vi "FFT-AxisVectorsFor2D.vi"(9 "Ny in":i32, 10 "Nx in":i32) -> (0 "Fy-Vector":dbl[](array[numeric]), 1 "Ny fft":i32, 2 "Fx Vector":dbl[](array[numeric]), 3 "Nx fft":i32)   [LabVIEW 2015]
uses:
  <vilib>/Analysis/1siggen.llb/Ramp Pattern by Delta.vi
  <vilib>/Analysis/NI_AALBase.lvlib
panel:
  in  "FFT shift?":bool=TRUE
  # "This creates so far only fake vector, but they have the same range and their length is correct"
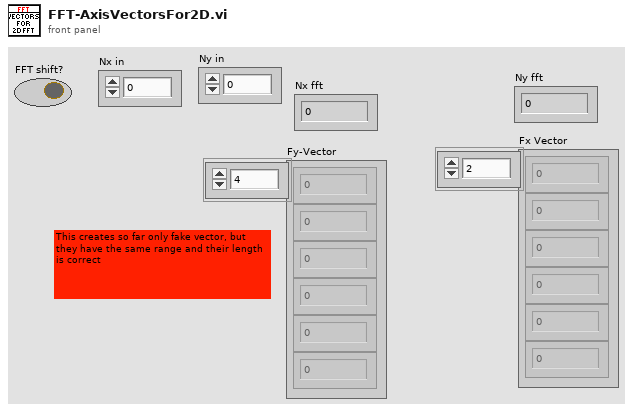
[diagram p1: front panel]
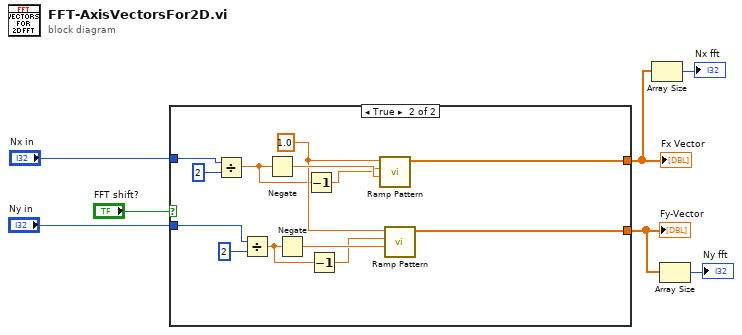
[diagram p0: block diagram]
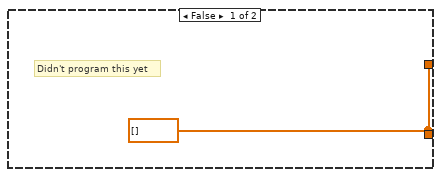
[diagram p2: hidden frame]
diagram:
  n1 = case shown="True" "FFT shift?" {
    tunnel: [w8 w21] -> w4
    tunnel: [w8 w20] -> w1
    tunnel: "Nx in" -> [_ w17]
    tunnel: "Ny in" -> [_ w19]
    frame False {
      w8 = dbl[] [] ("Ramp Pattern")
      # "Didn't program this yet"
    }
    frame True {
      w14 = 1.0 ("delta")
      n2 = Divide(x=w17, y=2) -> (x/y=w10:dbl)
      n3 = Divide(x=w19, y=2) -> (x/y=w12:dbl)
      n4 = Negate(x=w10) -> (-x=w15:dbl)
      n5 = Negate(x=w12) -> (-x=w13:dbl)
      n6 = Decrement(x=w10) -> (x-1=w9:dbl)
      n7 = Decrement(x=w12) -> (x-1=w11:dbl)
      n8 = call-poly <vilib>:"Ramp Pattern.vi"("start"=w15, "end"=w9, "delta"=w14) -> ("Ramp Pattern"=w21:dbl[])  [unwired: 6 in, 2 out]
      n9 = call-poly <vilib>:"Ramp Pattern.vi"("start"=w13, "end"=w11, "delta"=w14) -> ("Ramp Pattern"=w20:dbl[])  [unwired: 6 in, 2 out]
    }
  }
  "Fy-Vector" <- w1
  "Fx Vector" <- w4
  n10 = Array Size(array=w4) -> (size(s)=→"Nx fft":i32)
  n11 = Array Size(array=w1) -> (size(s)=→"Ny fft":i32)
